vi "Keyence.Main.Init.vi"(7 "Idx":i32, 8 "error in":errorcluster, 10 "restart":bool=TRUE, 11 "Data in":T1={"Status"={"State"=enum."Init", "Ref"=refnum, "Bank"=0, "Version"="", "Model"="", "EndTS"=timestamp(0 s since 1904-01-01), "ImgPath"=path ""}, "Sets"={"IP"="192.168.2.1", "Timeout_ms"=5000, "Retries"=0, "ReconnectPeriod_s"=0, "ResetPeriod_s"=0, "ReadImg"=FALSE}, "Code"={"text"="", "status"=FALSE, "corners"=[], "level"=0, "class"="", "path"=path ""}}) -> (0 "error out":errorcluster, 3 "Data out":T1={"Status"={"State"=enum."Init", "Ref"=refnum, "Bank"=0, "Version"="", "Model"="", "EndTS"=timestamp(0 s since 1904-01-01), "ImgPath"=path ""}, "Sets"={"IP"="192.168.2.1", "Timeout_ms"=5000, "Retries"=0, "ReconnectPeriod_s"=0, "ResetPeriod_s"=0, "ReadImg"=FALSE}, "Code"={"text"="", "status"=FALSE, "corners"=[], "level"=0, "class"="", "path"=path ""}})   [LabVIEW 2015]
uses:
  Keyence.Data.ctl
  Keyence.Data.Status.ctl
  Keyence.Data.Status.State.ctl
  Keyence.Data.Sets.ctl
  LowLevel/Keyence.CodeDetails.ctl
  LowLevel/Keyence.Global.vi
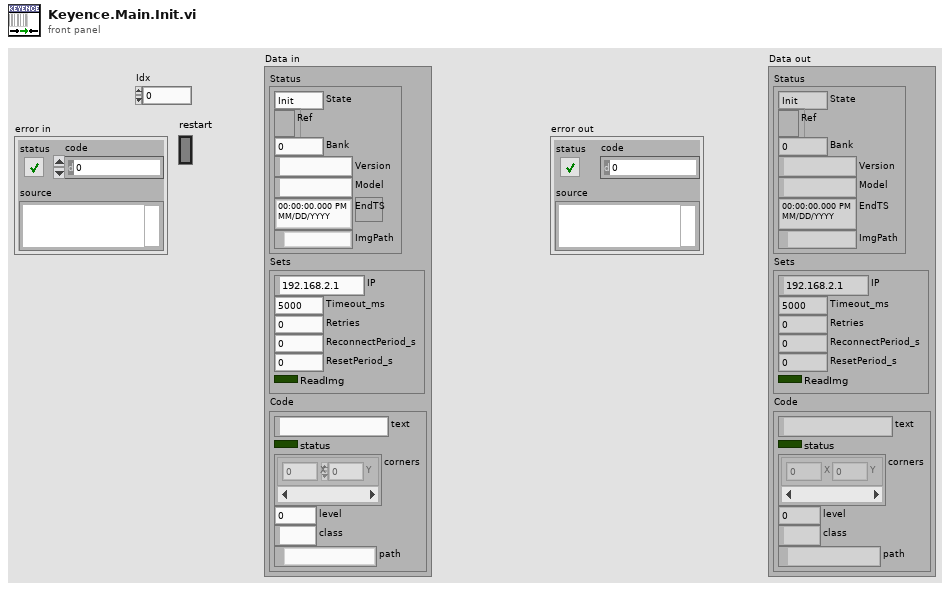
[diagram p1: front panel]
types:
  T1 = typedef "Keyence.Data.ctl" = cluster{"Status":T2, "Sets":T4, "Code":T5}
  T2 = typedef "Keyence.Data.Status.ctl" = cluster{"State":T3, "Ref":refnum<k5>, "Bank":u8, "Version":string, "Model":string, "EndTS":timestamp, "ImgPath":path}
  T3 = typedef "Keyence.Data.Status.State.ctl" = enum16{"First", "Init", "Reset", "Idle", "Scan"}
  T4 = typedef "Keyence.Data.Sets.ctl" = cluster{"IP":string, "Timeout_ms":i32, "Retries":i32, "ReconnectPeriod_s":i32, "ResetPeriod_s":i32, "ReadImg":bool}
  T5 = typedef "Keyence.CodeDetails.ctl" = cluster{"text":string, "status":bool, "corners":cluster{"X":i32, "Y":i32}[], "level":u8, "class":string, "path":path}
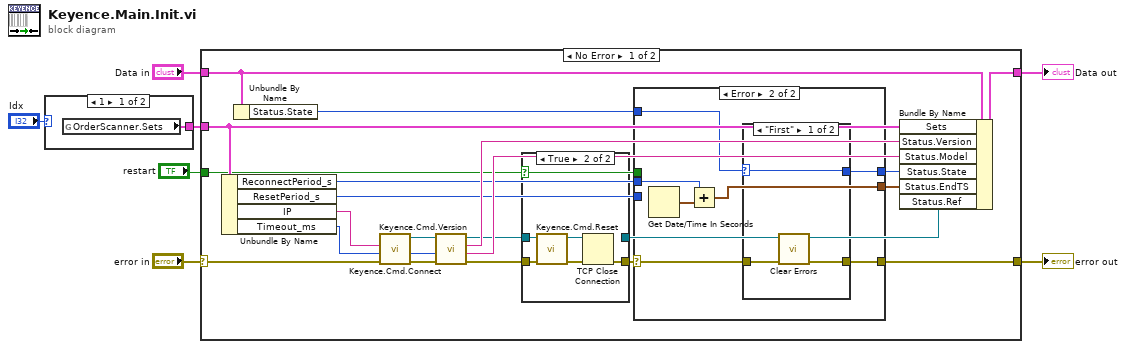
[diagram p0: block diagram]
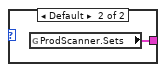
[diagram p2: hidden frame]
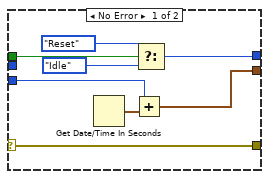
[diagram p4: hidden frame]
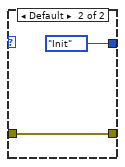
[diagram p5: hidden frame]
diagram:
  n1 = case shown="1" "Idx" {
    tunnel: [w8 w9] -> w3
    frame 1 {
      n2 = global read "Keyence.Global.vi" "OrderScanner.Sets"() -> (w8:T4)
    }
    frame Default {
      n3 = global read "Keyence.Global.vi" "ProdScanner.Sets"() -> (w9:T4)
    }
  }
  n4 = case shown="No Error" "error in" {
    selector: "error in" -> [w28 w59]
    tunnel: [w10 w59] -> w6
    tunnel: "Data in" -> [w12 w58]
    tunnel: [w30 w58] -> w4
    tunnel: w3 -> [w29 _]
    tunnel: "restart" -> [w14 _]
    frame No Error {
      n5 = Unbundle By Name(w29) -> ("ReconnectPeriod_s"=w16:i32, "ResetPeriod_s"=w17:i32, "IP"=w25:string, "Timeout_ms"=w26:i32)
      n6 = Unbundle By Name(w12) -> ("Status.State"=w11:T3)
      n7 = call "Keyence.Cmd.Connect.vi"("error in (no error)"=w28, "Timeout [ms] (1000)"=w26, "IP"=w25) -> ("error out"=w27:errorcluster, "connection ID out"=w24:refnum<k5>)  [unwired: 7 in]
      n8 = call "Keyence.Cmd.Version.vi"("error in (no error)"=w27, "Timeout [ms] (1000)"=w26, "connection ID"=w24) -> ("error out"=w21:errorcluster, "version"=w22:string, "model"=w23:string, "connection ID out"=w19:refnum<k5>)  [unwired: 4 in, 1 out]
      n9 = case shown="True" w14 {
        tunnel: w21 -> [w32 w37]
        tunnel: w19 -> [w31 w36]
        tunnel: [w32 w33] -> w18
        tunnel: [w31 _] -> w13
        frame False {
        }
        frame True {
          n10 = call "Keyence.Cmd.Reset.vi"("error in (no error)"=w37, "connection ID"=w36) -> ("error out"=w34:errorcluster, "connection ID out"=w35:refnum<k5>)  [unwired: 8 in]
          n11 = TCP Close Connection(connection ID=w35, error in (no error)=w34) -> (error out=w33:errorcluster)  [unwired: 1 in, 1 out]
        }
      }
      n12 = case shown="Error" w18 {
        selector: w18 -> [w38 w47]
        tunnel: [w41 w52] -> w20
        tunnel: w17 -> [w44 _]
        tunnel: w16 -> [_ w51]
        tunnel: [w43 w49] -> w15
        tunnel: w14 -> [w39 _]
        tunnel: w11 -> [_ w48]
        tunnel: [w38 w46] -> w10
        frame No Error {
          n13 = Get Date/Time In Seconds() -> (seconds since 1Jan1904=w45:timestamp)
          n14 = Add(x=w44, y=w45) -> (x+y=w43:timestamp)
          n15 = Select(t=Keyence.Data.Status.State."Reset" ("Status.State"), s=w39, f=Keyence.Data.Status.State."Idle" ("Status.State")) -> (s? t:f=w41:T3)
        }
        frame Error {
          n16 = Get Date/Time In Seconds() -> (seconds since 1Jan1904=w50:timestamp)
          n17 = Add(x=w51, y=w50) -> (x+y=w49:timestamp)
          n18 = case shown="\"First\"" w48 {
            selector: w48 -> [w55 _]
            tunnel: [w55 Keyence.Data.Status.State."Init" ("Status.State")] -> w52
            tunnel: w47 -> [w54 w56]
            tunnel: [w53 w56] -> w46
            frame "First" {
              n19 = call <vilib>:"Clear Errors.vi"("error in (no error)"=w54) -> ("error out"=w53:errorcluster)  [unwired: 5 in, 1 out]
            }
            frame Default {
            }
          }
        }
      }
      n20 = Bundle By Name(cluster=w12, "Sets"=w29, "Status.Version"=w23, "Status.Model"=w22, "Status.State"=w20, "Status.EndTS"=w15, "Status.Ref"=w13) -> (w30:T1)
    }
    frame Error {
    }
  }
  "error out" <- w6
  "Data out" <- w4
